vi "RT_DAC_ADC_voltage_WnR.vi"() -> ()   [LabVIEW 2018]
uses:
  <vilib>/rvi/interface/nirviOpenFPGA/nirviOpenFPGA.xnode
  <vilib>/rvi/interface/nirviReadWriteControl/nirviReadWriteControl.xnode
  NiFpgaLv.dll
  <vilib>/Utility/error.llb/Error Cluster From Error Code.vi
  <vilib>/rvi/interface/Simulation/niFpgaSimulationCallBeginRW.vi
  <vilib>/rvi/errors/niLvFpgaAdjustHostInterfaceError.vi
  FPGA Bitfiles/ASPE2019amplifie_FPGATarget_fpga1DACsineand1_1p-Bv2BD-MI.lvbitx
  FPGA files/fpga_1DAC_sine_and_1ADC_W_risingedge_R_trailingedge_stacked.vi
  <vilib>/FPGAPlugInAG/myRIO-1900/niLvFpga_Open_myRIO-1900.vi
  <vilib>/rvi/interface/common/dynamic/niFpgaDynamicAddResources.vi
panel:
  in  "voltage":dbl
  in  "Stop Button":bool
  out "Waveform Chart 4":dbl(graph)
  out "Waveform Chart 3":dbl(graph)
  out "Waveform Chart 2":dbl(graph)
  out "Waveform Chart":dbl(graph)=0.00366205349649816
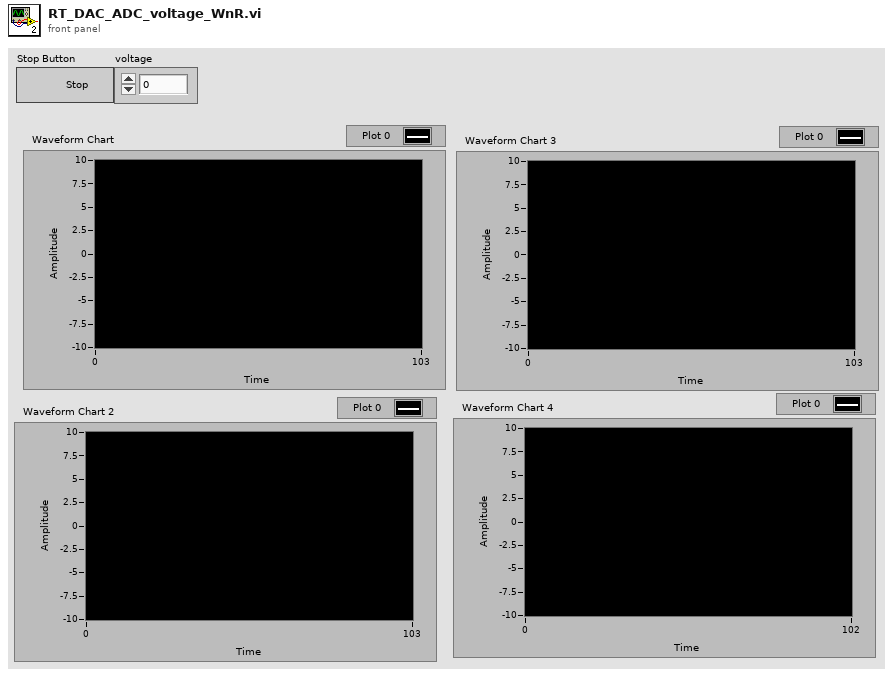
[diagram p1: front panel]
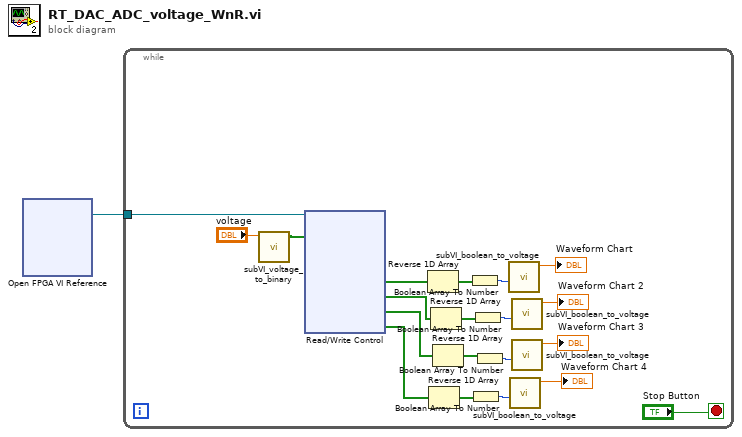
[diagram p0: block diagram]
diagram:
  n1 = xnode "Open FPGA VI Reference"() -> ("FPGA VI Reference Out"=w1:refnum<k20>)  [unwired: 2 in, 1 out]
  n2 = while {
    tunnel: w1 -> [w21]
    stop <- "Stop Button" stop-if-true
    n3 = call "subVI_voltage_to_binary.vi"("voltage"="voltage") -> ("binary"=w3:bool[])  [unwired: 10 in]
    n4 = xnode "Read/Write Control"("FPGA VI Reference In"=w21, "DAC 1 write"=w3) -> ("ADC1 read"=w19:bool[], "ADC2 read"=w15:bool[], "ADC3 read"=w12:bool[], "ADC3 read"=w9:bool[])  [unwired: 3 in, 2 out]
    n5 = Reverse 1D Array(array=w19) -> (reversed array=w20:bool[])
    n6 = Reverse 1D Array(array=w9) -> (reversed array=w11:bool[])
    n7 = Reverse 1D Array(array=w15) -> (reversed array=w17:bool[])
    n8 = Reverse 1D Array(array=w12) -> (reversed array=w14:bool[])
    n9 = Boolean Array To Number(Boolean array=w20) -> (number=w18:u16)
    n10 = Boolean Array To Number(Boolean array=w11) -> (number=w10:u16)
    n11 = Boolean Array To Number(Boolean array=w17) -> (number=w16:u16)
    n12 = Boolean Array To Number(Boolean array=w14) -> (number=w13:u16)
    n13 = call "subVI_boolean_to_voltage.vi"(9:w18) -> ("V"=→"Waveform Chart":dbl)  [unwired: 10 in]
    n14 = call "subVI_boolean_to_voltage.vi"(9:w10) -> ("V"=→"Waveform Chart 4":dbl)  [unwired: 10 in]
    n15 = call "subVI_boolean_to_voltage.vi"(9:w16) -> ("V"=→"Waveform Chart 2":dbl)  [unwired: 10 in]
    n16 = call "subVI_boolean_to_voltage.vi"(9:w13) -> ("V"=→"Waveform Chart 3":dbl)  [unwired: 10 in]
  }
